vi "Measure Voltage.vi"(8 "error in (no error)":errorcluster, 11 "VISA name":refnum<visa-resource-name>="GPIB::5::INSTR") -> (0 "error out":errorcluster, 2 "Output Voltage [V]":dbl format="%.4f")   [LabVIEW 2020, in "Low Level PSU With Tests.lvlib"]
uses:
  VISA/VISA Instrument.lvclass
  C:/Git/astemes-gdevcon-2022/PSU Demo/Low Level PSU With Tests/Instrument Interface/Instrument.lvclass
  Low Level PSU With Tests.lvlib
  Low Level PSU/Low Level PSU.lvclass
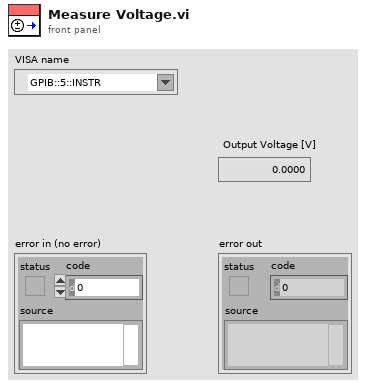
[diagram p1: front panel]
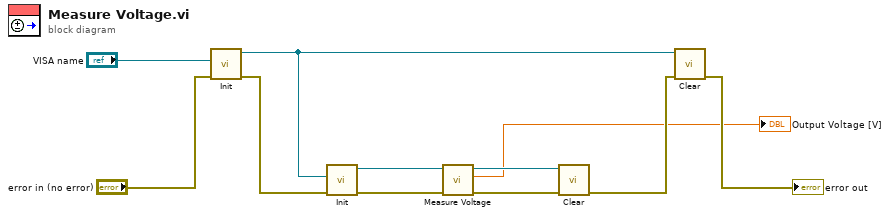
[diagram p0: block diagram]
diagram:
  n1 = call "Init.vi"("error in (no error)"="error in (no error)", "VISA name"="VISA name") -> ("error out"=w6:errorcluster, "VISA out"=w2:refnum<class "VISA Instrument.lvclass">)  [unwired: 8 in]
  n2 = call "Init.vi"("error in (no error)"=w6, "Instrument Interface"=w2) -> ("error out"=w10:errorcluster, "Low Level PSU Out"=w11:refnum<class "Low Level PSU.lvclass">)  [unwired: 8 in]
  n3 = call "Measure Voltage.vi"("error in (no error)"=w10, "Low Level PSU In"=w11) -> ("error out"=w8:errorcluster, "Output Voltage"=→"Output Voltage [V]":dbl, "Low Level PSU Out"=w9:refnum<class "Low Level PSU.lvclass">)  [unwired: 7 in]
  n4 = call "Clear.vi"("error in (no error)"=w8, "Low Level PSU In"=w9) -> ("error out"=w5:errorcluster)  [unwired: 8 in, 1 out]
  n5 = call "Clear.vi"("error in (no error)"=w5, "VISA in"=w2) -> ("error out"=→"error out":errorcluster)  [unwired: 8 in, 1 out]
